vi "Bertta_v08_2.vi"() -> ()   [LabVIEW 2015]
panel:
  out "Started:":string
  in  "SHUTDOWN":bool
  in  "MASTER CONTROL":bool
  in  "Tab Control":T1(tab)
  in  "Read Seq":bool
  in  "Save Seq":bool
  in  "Configuration file":path=path "C:/Users/shresplab/Desktop/BerttaConfiguration.lvm" caption="Filename"
  in  "OK Button 2":bool
  out "Boolean":bool
  in  "User (initials)":string
  in  "Project name":string
  in  "Description":string
  out "Output file":string
  in  "OK Button":bool
  in  "Add comment":string
  out "PUMP 1":bool
  out "Target amount":dbl
  out "Scale weight":dbl
  out "Amount now":dbl
  out "Flow rate":dbl
  out "Time to target":dbl format="%<%H:%M:%S>t"
  out "Current step":dbl
  out "Target amount":dbl
  out "Amount now":dbl
  out "Tr":dbl
  out "Tj in":dbl
  out "Tj out":dbl
  out "T set":dbl
  out "Current step":i32
  out "RPM":dbl
  out "Torque 2":dbl
  out "Waveform Chart 5":dynamicdata(graph)
  out "Waveform Chart 6":dynamicdata(graph)
  out "Waveform Chart 7":dynamicdata(graph)
  in  "Tab Control 2":T2(tab)
  out "Waveform Chart 3":dynamicdata(graph)
  out "Waveform Chart 8":dynamicdata(graph)
  out "Waveform Chart 9":dynamicdata(graph)
  out "Table":string[][](table)=[["Date / time", "Flow rate, P1, g/min", "Weight, S1, g", "Amount / step, P1, g", "Step number, P1", "Total amount,P1, g ", "Tj in, C", "Tj out, C", "Tr, C", "RPM", "Torque", ""], ["11.8.2017 13.29.21", "0,000000", "423,900000", "-423,900000", "1,000000", "20,000000", "22,722972", "22,704167", "22,605956", "0,000000", "395,000000", "4,800000"], ["11.8.2017 13.29.26", "0,000000", "423,900000", "0,000000", "1,000000", "20,000000", "22,719822", "22,702434", "22,603119", "0,000000", "0,000000", "0,000000"], ["11.8.2017 13.29.31", "0,000000", "423,900000", "0,000000", "1,000000", "20,000000", "22,719034", "22,702118", "22,600441", "0,000000", "0,000000", "0,000000"], ["11.8.2017 13.29.37", "0,000000", "423,900000", "0,000000", "1,000000", "20,000000", "22,717459", "22,701015", "22,596344", "0,000000", "63,000000", "2,600000"], ["11.8.2017 13.29.42", "0,000000", "423,900000", "0,000000", "1,000000", "20,000000", "22,716829", "22,699440", "22,595242", "0,000000", "199,000000", "3,900000"], ["11.8.2017 13.29.47", "0,000000", "423,900000", "0,000000", "1,000000", "20,000000", "22,715411", "22,699282", "22,593351", "0,000000", "269,000000", "4,300000"], ["11.8.2017 13.29.52", "0,000000", "423,900000", "0,000000", "1,000000", "20,000000", "22,714466", "22,698967", "22,588624", "0,000000", "300,000000", "4,300000"], ["11.8.2017 13.29.58", "0,000000", "423,900000", "0,000000", "1,000000", "20,000000", "22,712733", "22,697234", "22,586261", "0,000000", "300,000000", "4,300000"], ["11.8.2017 13.30.03", "0,000000", "423,900000", "0,000000", "1,000000", "20,000000", "22,710370", "22,696604", "22,585315", "0,000000", "300,000000", "4,400000"], ["11.8.2017 13.30.08", "0,000000", "424,100000", "-0,200000", "1,000000", "20,000000", "22,709425", "22,696131", "22,583582", "0,000000", "300,000000", "4,300000"], ["11.8.2017 13.30.13", "0,000000", "424,200000", "-0,300000", "1,000000", "20,000000", "22,708008", "22,693925", "22,582952", "0,000000", "300,000000", "0,000000"], ["11.8.2017 13.30.18", "0,000000", "424,200000", "-0,300000", "1,000000", "20,000000", "22,706117", "22,693453", "22,583740", "0,000000", "300,000000", "4,300000"], ["11.8.2017 13.30.23", "0,000000", "424,200000", "-0,300000", "1,000000", "20,000000", "22,706747", "22,693768", "22,587048", "0,000000", "300,000000", "4,400000"], ["11.8.2017 13.30.28", "0,000000", "424,200000", "-0,300000", "1,000000", "20,000000", "22,706275", "22,694556", "22,590357", "0,000000", "300,000000", "39,100000"], ["11.8.2017 13.30.33", "0,000000", "424,200000", "-0,300000", "1,000000", "20,000000", "22,705645", "22,693925", "22,594296", "0,000000", "300,000000", "5,300000"]]
  in  "T ext / T ext 2":enum32{"External 1", "External 2"}(radio)
  out "Sensor OK":bool
  in  "T fail":dbl=20.0
  out "Boolean 12":bool
  out "Boolean 7":bool
  out "Boolean 6":bool
  out "Boolean 5":bool
  out "Boolean 4":bool
  in  "?":bool
  in  "T setpoint":dbl=20.0
  in  "Lauda port":dbl=9.0
  out "Data out":dbl
  in  "Bypass select":enum32{"Tr", "Tj"}(radio)
  in  "TempSeq":dbl[][](array[numeric])=[[20.0, 45.0, 50.0, 46.0], [46.0, 50.0, 20.0, 51.0], [20.0, 50.0, 3.0, 25.0], [20.0, 20.0, 0.0, 20.0], [20.0, 20.0, 0.0, 20.0], [20.0, 20.0, 1000.0, 20.0]]
  out "T control":dbl
  out "Tr":dbl
  out "Tj in":dbl
  out "Tj out":dbl
  out "DT":dbl
  out "Elapsed":i32
  in  "PAUSE":bool
  out "Boolean 19":bool
  in  "Reset":bool
  in  "Treshold (Tset)":dbl=1.0
  in  "Tmax":dbl=140.0
  in  "Tmin":dbl=20.0
  out "Current step":i32
  out "Tset":dbl
  out "Waveform Chart":dynamicdata(graph)
  out "T external 2":dbl
  in  "Ring":u16(ring) items=["SCALE 1", "SCALE 2", "SCALE 3"]
  out "Data out":dbl
  out "Port":i32=10
  in  "Radio Buttons":enum32{"Reglo Digital", "Reglo Analog", "PAM"}(radio)
  out "Speed":dbl
  out "mA":dbl format="%#_2g"
  in  "Port":i32=15
  out "RPM":dbl format="%#_2g"
  out "Boolean 18":bool
  out "Boolean 17":bool
  out "Boolean 16":bool
  out "Boolean 15":bool
  out "Boolean 14":bool
  out "Boolean 13":bool
  out "Boolean 11":bool
  out "Boolean 10":bool
  out "Boolean 9":bool
  out "Boolean 8":bool
  in  "PumpSeq":dbl[][](array[numeric])=[[3.0, 3.0, 7.0], [2.0, 2.0, 2.0], [4.0, 2.0, 100.0], [0.0, 0.0, 0.0], [0.0, 0.0, 0.0], [0.0, 0.0, 0.0], [0.0, 0.0, 0.0], [0.0, 0.0, 0.0], [0.0, 0.0, 0.0], [0.0, 0.0, 0.0], [0.0, 1.0, 0.0]]
  in  "?":bool
  out "Flow rate (g/min)":dbl
  out "Time (min)":dbl
  out "Target (g)":dbl
  out "Scale reading":dbl
  out "Step amount now":dbl
  out "Time to target":dbl format="%<%H:%M:%S>t"
  in  "Grams / min":dbl
  out "Waveform Chart 2":dynamicdata(graph)
  in  "?":bool
  out "Total amount now":dbl
  out "Total time":dbl
  out "Total amount target":dbl
  out "Boolean 20":bool
  in  "Reset 2":bool
  in  "Bypass select 2":enum32{"Remote", "Manual"}(radio)
  in  "Port":dbl=13.0
  out "RPM":dbl
  out "Torque":dbl
  in  "Set RPM":dbl(slide) scale=0.0..500.0
  out "Waveform Chart 4":dynamicdata(graph)
  out "DAQ 9217 (PT100)":errorcluster
  # "PUMP & SCALE 1"
  # "STEP"
  # "TOTAL"
  # "Tinit     >    Tset       Min. time      Tfail"
  # "Manual control / end of sequence"
  # "Manual control"
  # "Secondary temperature sensor"
  # "Device communication"
  # "Grams    /   min"
  # "End of sequence"
  # "Manual control"
  # "Device communication"
  # "Pump configuration"
  # "Scale configuration"
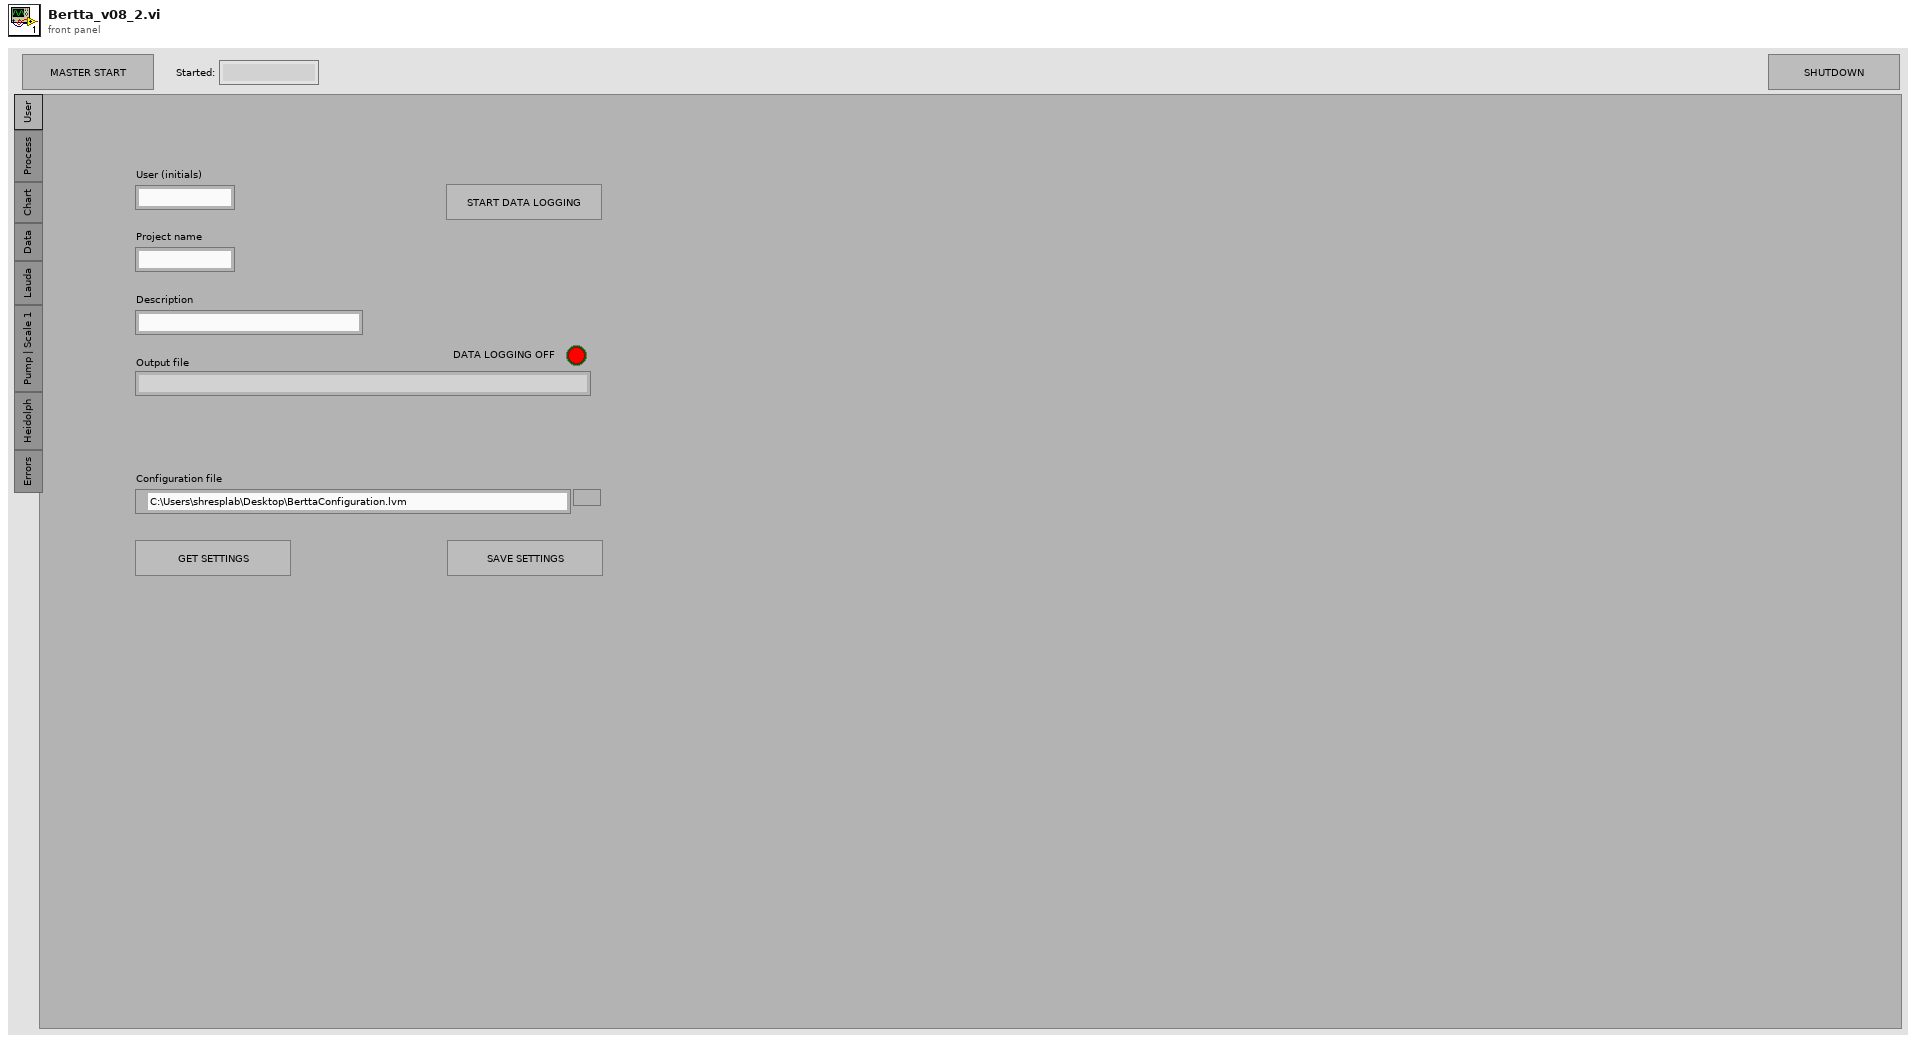
[diagram p1: front panel]
types:
  T1 = enum32{"User", "Process", "Chart", "Data", "Lauda", "Pump | Scale 1", "Heidolph", "Errors"}
  T2 = enum32{"Temperatures", "Scale / Pump 1", "RPM / torque"}
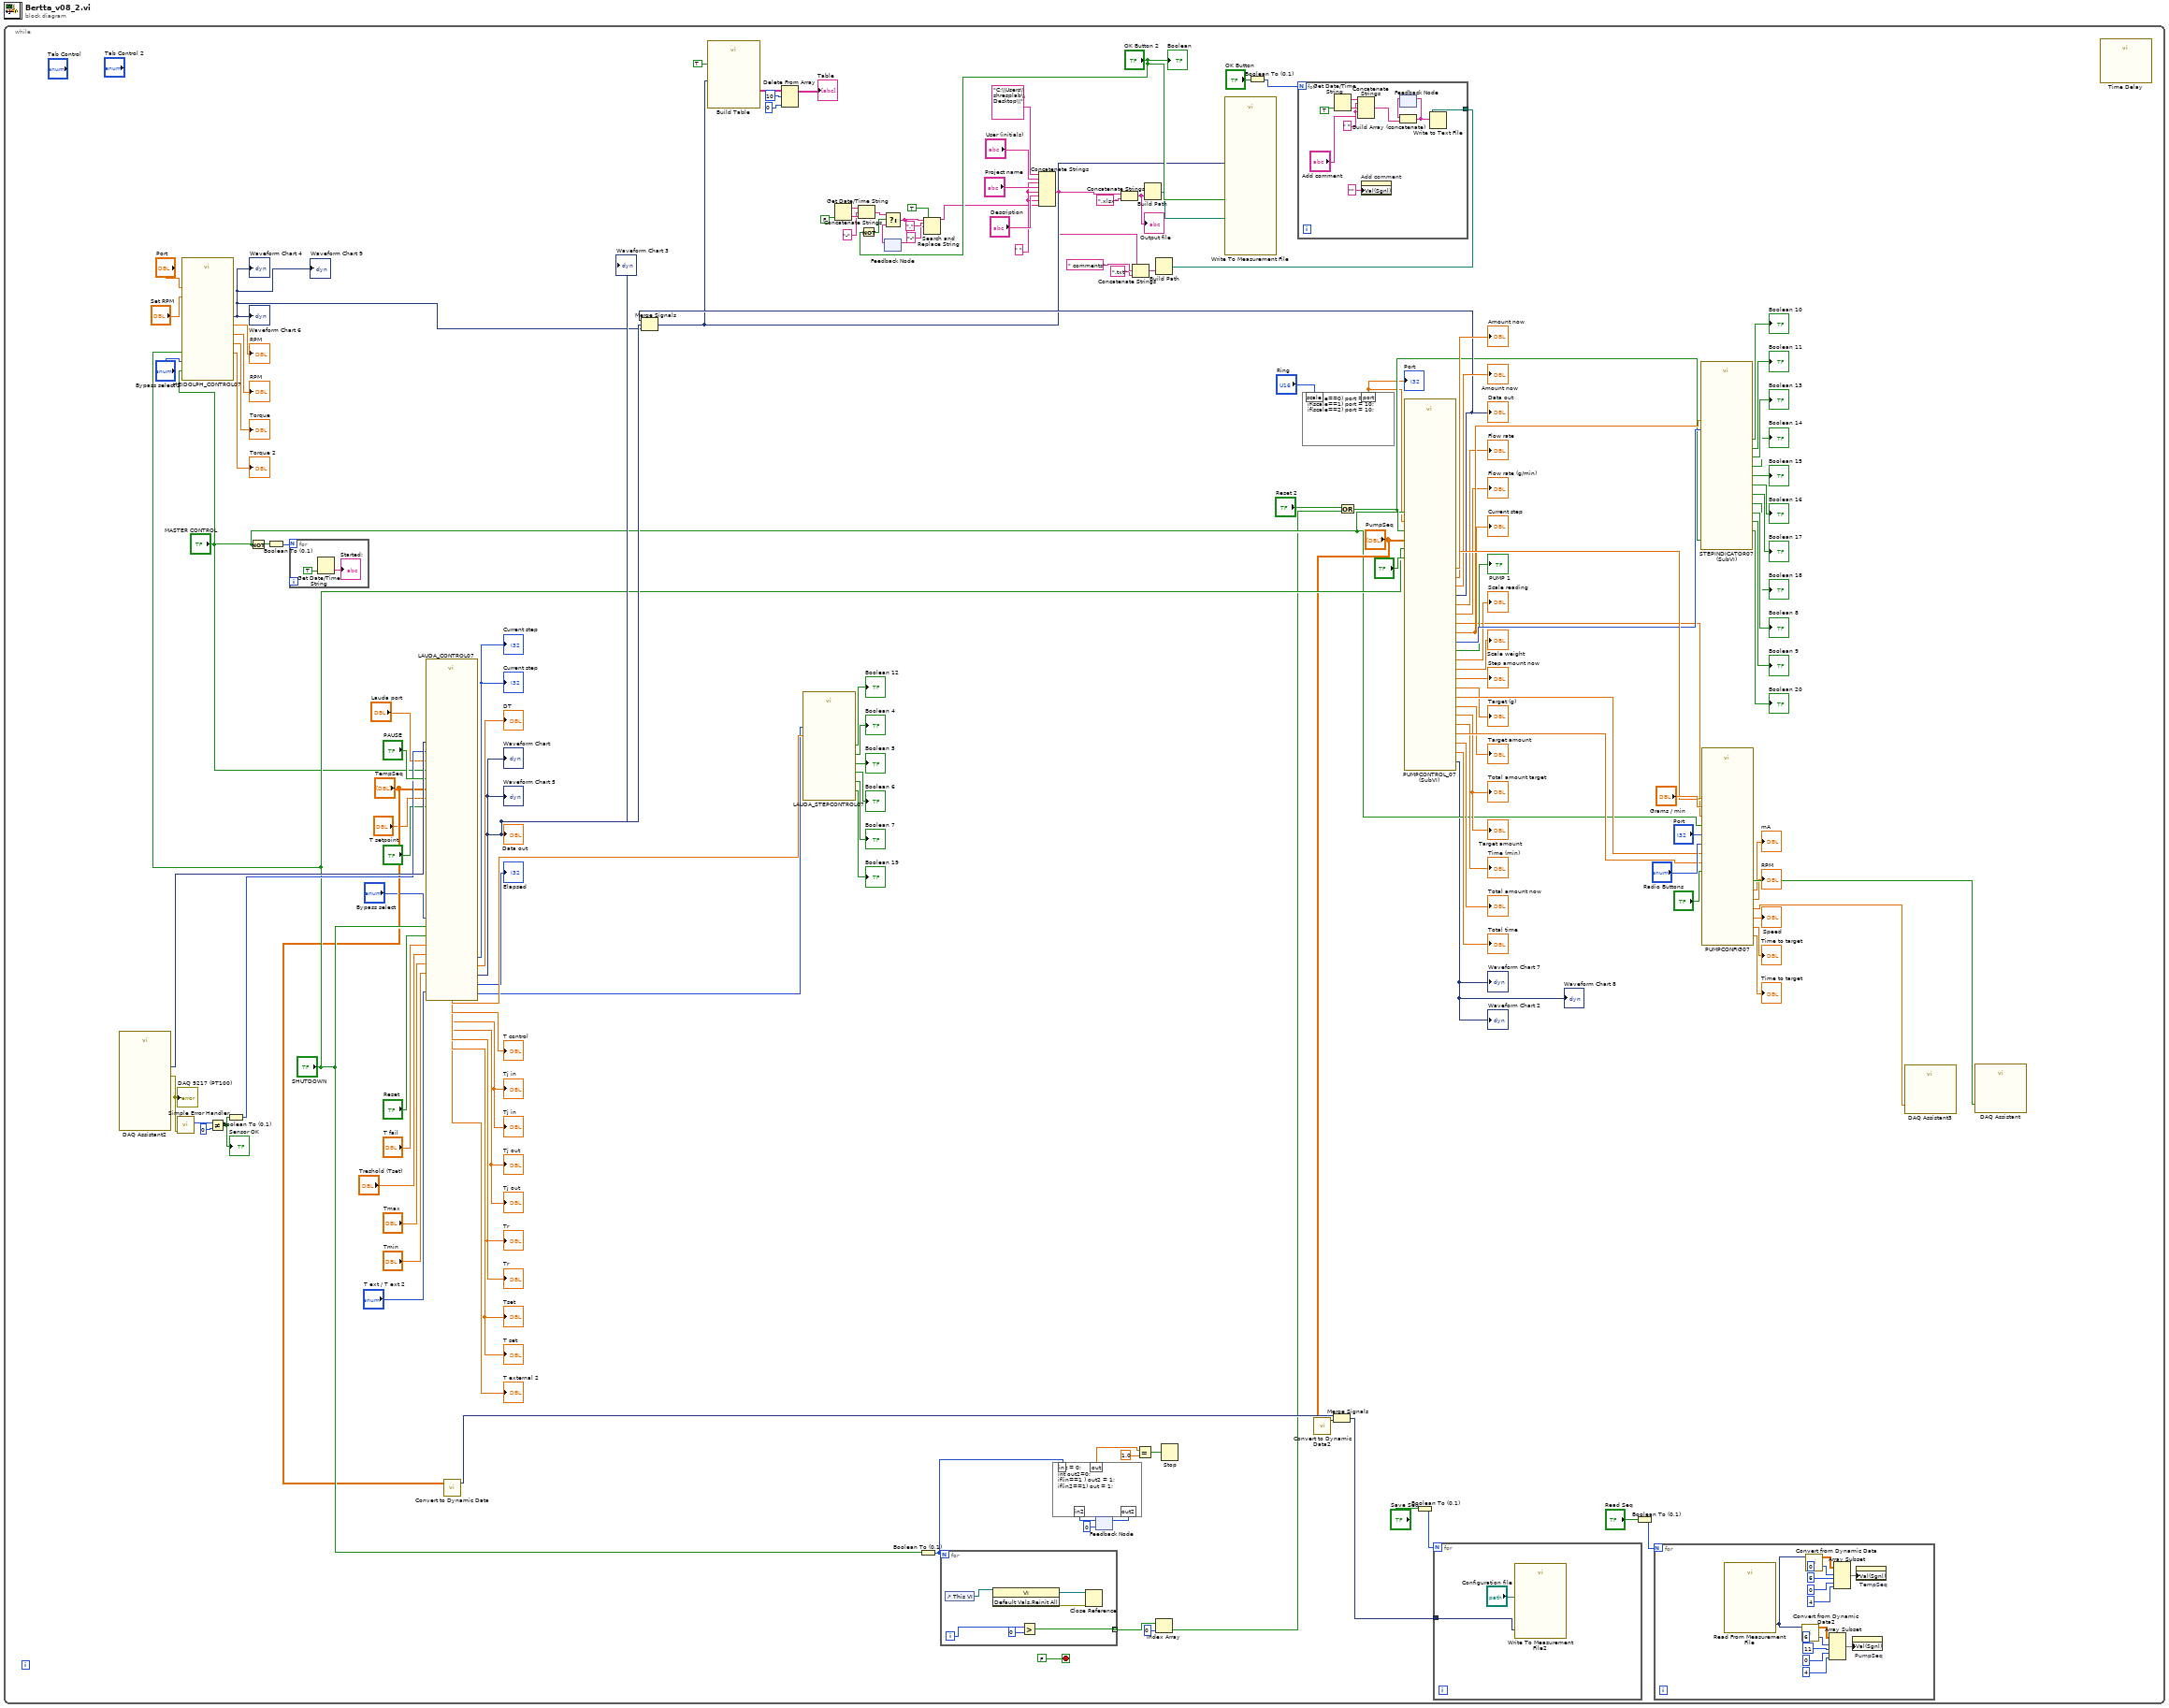
[diagram p0: block diagram]
diagram:
  n1 = while {
    stop <- FALSE stop-if-true
    w81 = " "
    n2 = call "DAQ Assistant2"() -> ("data"=w144:dynamicdata, "error out"=w88:errorcluster)  [unwired: 17 in, 1 out]
    "DAQ 9217 (PT100)" <- w88
    n3 = call <vilib>:"Simple Error Handler.vi"("error in (no error)"=w88) -> ("code out"=w87:i32)  [unwired: 4 in, 4 out]
    n4 = call "HEIDOLPH_CONTROL07.vi"("master"="MASTER CONTROL", "shutdown"="SHUTDOWN", "Bypass select"="Bypass select 2", "Set RPM"="Set RPM", "Device port"="Port") -> ("Dynamic Data"=w93:dynamicdata, "RPM"=→"RPM":dbl, "RPM 2"=→"RPM":dbl, "Torque"=→"Torque":dbl, "Torque 2"=→"Torque 2":dbl)  [unwired: 2 in]
    "Waveform Chart 4" <- w93
    "Waveform Chart 6" <- w93
    "Waveform Chart 9" <- w93
    n5 = Not Equal?(x=w87, y=0) -> (x != y?=w51:bool)
    "Sensor OK" <- w51
    n6 = Boolean To (0,1)(Boolean=w51) -> (0, 1=w85:i16)
    n7 = Not(x="MASTER CONTROL") -> (.not. x?=w69:bool)
    n8 = Boolean To (0,1)(Boolean=w69) -> (0, 1=w70:i16)
    n9 = for {
      N: w70 -> [_]
      n10 = Get Date/Time String(want seconds? (F)=TRUE) -> (time string=→"Started:":string)  [unwired: 2 in, 1 out]
    }
    n11 = call "LAUDA_CONTROL07.vi"("Bypass"="?", "PAUSE"="PAUSE", "data"=w144, "Seq"="TempSeq", "Lauda port"="Lauda port", "Tbypass"="T setpoint", "Treshold"="Treshold (Tset)", "Bypass select"="Bypass select", "err"=w85, "Shutdown"="SHUTDOWN", "Master Start"="MASTER CONTROL", "Reset"="Reset", "Tfail (manual)"="T fail", "Tmax"="Tmax", "T ext / T ext 2"="T ext / T ext 2", "Tmin"="Tmin") -> ("Tj in"=→"Tj in" →"Tj in":dbl, "DT"=→"DT":dbl, "Tj out"=→"Tj out" →"Tj out":dbl, "Tset"=→"Tset" →"T set":dbl, "Dynamic Data"=w95:dynamicdata, "T ext 2"=→"T external 2":dbl, "Numeric"=w73:i16, "Numeric 2"=w149:dbl, "T control"=→"T control":dbl, "Current step"=→"Current step" →"Current step":i32, "Elapsed"=→"Elapsed":i32, "Tr"=→"Tr" →"Tr":dbl)
    "Waveform Chart 3" <- w95
    "Waveform Chart" <- w95
    "Data out" <- w95
    "Waveform Chart 5" <- w95
    n12 = call "Convert to Dynamic Data"("2D Array"="TempSeq") -> ("Dynamic Data Type"=w61:dynamicdata)  [unwired: 3 in]
    n13 = call "LAUDA_STEPCONTROL07.vi"("Numeric 2"=w149, "Numeric"=w73) -> ("Boolean 13"=→"Boolean 19":bool, "Boolean 6"=→"Boolean 6":bool, "Boolean 5"=→"Boolean 5":bool, "Boolean 4"=→"Boolean 4":bool, "Boolean 7"=→"Boolean 7":bool, "Boolean 12"=→"Boolean 12":bool)  [unwired: 4 in]
    n14 = Get Date/Time String(want seconds? (F)=FALSE) -> (date string=w35:string, time string=w30:string)  [unwired: 2 in]
    n15 = Concatenate Strings(w35, "-" ("string"), w30) -> (w34:string)
    n16 = Not(x="OK Button 2") -> (.not. x?=w31:bool)
    n17 = feedback #1() -> (w33:string)  [unwired: 1 in]
    n18 = Select(t=w34, s=w31, f=w33) -> (s? t:f=w26:string)
    n19 = feedback-in #1(w26) -> ()
    n20 = Boolean To (0,1)(Boolean="SHUTDOWN") -> (0, 1=w4:i16)
    n21 = Search and Replace String(replace all?=TRUE ("replace all? (F)"), input string=w26, search string=".", replace string="-" ("replace string (\"\")")) -> (result string=w25:string)  [unwired: 4 in, 3 out]
    n22 = for {
      N: w4 -> [_]
      tunnel: [w176] -> w64 mode=indexing
      i -> [w178]
      n23 = control-ref of="This VI"() -> (w181:refnum<vi>)
      n24 = invoke class="VI" method="Default Vals.Reinit All"(reference=w181) -> (reference out=w179:refnum<vi>, error out=w180:errorcluster)  [unwired: 2 in, 1 out]
      n25 = Greater?(x=w178, y=0) -> (0:w176:bool)
      n26 = Close Reference(reference=w179, error in (no error)=w180) -> ()  [unwired: 1 out]
    }
    n27 = Concatenate Strings("C:\\Users\\shresplab\\Desktop\\", "User (initials)", w81, "Project name", w81, "Description", w81, w25) -> (w15:string)
    n28 = feedback #2(0) -> (w2:i32)
    n29 = formula code="out = 0;\nint out2=0;\nif(in==1 ) out2 = 1;\nif(in2==1) out = 1;"("in"=w4, "in2"=w2) -> ("out"=w7:dbl, "out2"=w3:i32)
    n30 = feedback-in #2(w3) -> ()
    n31 = Concatenate Strings(w15, ".xlsx") -> (w18:string)
    "Output file" <- w18
    n32 = Concatenate Strings(w15, " comments" ("string"), ".txt" ("string")) -> (w12:string)
    n33 = Equal?(x=w7, y=1.0) -> (x = y?=w6:bool)
    n34 = Build Path(name or relative path=w18) -> (appended path=w16:path)  [unwired: 1 in]
    n35 = Index Array(array=w64, index=0) -> (element=w5:bool)
    n36 = Build Path(name or relative path=w12) -> (appended path=w11:path)  [unwired: 1 in]
    n37 = Stop(stop? (T)=w6) -> ()
    n38 = Boolean To (0,1)(Boolean="OK Button") -> (0, 1=w10:i16)
    n39 = for {
      N: w10 -> [_]
      tunnel: w11 -> [w153]
      w157 = " " ("string")
      n40 = Get Date/Time String(want seconds? (F)=TRUE) -> (date string=w160:string, time string=w158:string)  [unwired: 2 in]
      n41 = Concatenate Strings(w160, w157, w158, w157, "Add comment") -> (w156:string)
      n42 = property on="Add comment" class="Str"("Val(Sgnl)"="" ("Value (Signaling)")) -> ()  [unwired: 2 in, 2 out]
      n43 = feedback #3() -> (w155:string[])  [unwired: 1 in]
      n44 = Build Array (concatenate)(w155, w156) -> (w154:string[])
      n45 = feedback-in #3(w154) -> ()
      n46 = Write to Text File(file (use dialog)=w153, text=w154) -> ()  [unwired: 2 in, 3 out]
    }
    n47 = formula code="if(scale==0) port = 10;\nif(scale==1) port = 10;\nif(scale==2) port = 10;"("scale"="Ring") -> ("port"=w39:dbl)
    "Port" <- w39
    n48 = call "Convert to Dynamic Data2"("2D Array"="PumpSeq") -> ("Dynamic Data Type"=w59:dynamicdata)  [unwired: 3 in]
    n49 = Merge Signals(w61, w59) -> (w58:dynamicdata)
    n50 = Or(x="Reset 2", y=w5) -> (x .or. y?=w50:bool)
    n51 = call "PUMPCONTROL_07 (SubVI).vi"("Port"=w39, "Pause"="MASTER CONTROL", "Master start"="?", "shutdown"="SHUTDOWN", "Seq in"="PumpSeq", "reset"=w50) -> ("Amount now"=→"Amount now":dbl, "Amount now 2"=→"Amount now":dbl, "Flow rate out"=w76:dbl, "Step amount now"=→"Step amount now":dbl, "Total amount now"=→"Total amount now":dbl, "Total time"=→"Total time":dbl, "Numeric 2"=w140:i16, "PUMP 1"=→"PUMP 1":bool, "Numeric"=w136:dbl, "Flow rate"=→"Flow rate":dbl, "Dynamic Data"=w94:dynamicdata, "Target amount"=→"Target amount":dbl, "Time (min) 2"=w141:dbl, "Target amount 2"=→"Total amount target" →"Target amount":dbl, "Scale reading"=→"Scale reading":dbl, "Flow rate (g/min)"=→"Flow rate (g/min)":dbl, "Target (g) 2"=w142:dbl, "Target (g)"=→"Target (g)":dbl, "Time (min)"=→"Time (min)":dbl, "Waveform Chart 2"=→"Waveform Chart 2" →"Waveform Chart 7" →"Waveform Chart 8":dynamicdata, "Scale weight"=→"Scale weight":dbl, "Amount (g)"=w143:dbl)
    "Current step" <- w136
    "Data out" <- w94
    n52 = Merge Signals(w94, w95, w93) -> (w22:dynamicdata)
    n53 = call "Build Table"("Include time data"=TRUE, "Signals"=w22) -> ("Table"=w21:string[][])  [unwired: 3 in, 6 out]
    n54 = Delete From Array(array=w21, length=10, index (col)=0 ("index (row)")) -> (array with subset deleted=→"Table":string[][])  [unwired: 1 in, 1 out]
    n55 = call "Write To Measurement File"("Signals"=w22, "Enable"="OK Button 2", "Filename"=w16) -> ()  [unwired: 14 in, 3 out]
    n56 = Boolean To (0,1)(Boolean="Save Seq") -> (0, 1=w57:i16)
    n57 = for {
      N: w57 -> [_]
      tunnel: w58 -> [w175]
      n58 = call "Write To Measurement File2"("Signals"=w175, "Filename"="Configuration file") -> ()  [unwired: 15 in, 3 out]
    }
    n59 = Boolean To (0,1)(Boolean="Read Seq") -> (0, 1=w54:i16)
    n60 = for {
      N: w54 -> [_]
      n61 = call "Read From Measurement File"() -> ("Signals"=w163:dynamicdata)  [unwired: 6 in, 5 out]
      n62 = call "Convert from Dynamic Data2"("Dynamic Data Type"=w163) -> ("Array"=w162:dbl[][])  [unwired: 3 in]
      n63 = call "Convert from Dynamic Data"("Dynamic Data Type"=w163) -> ("Array"=w171:dbl[][])  [unwired: 3 in]
      n64 = Array Subset(array=w162, index (row)=6 ("index"), length (row)=11 ("length"), index (col)=0 ("index"), length (col)=4 ("length")) -> (w161:dbl[][])
      n65 = Array Subset(array=w171, index (row)=0 ("index"), length (row)=6 ("length"), index (col)=0 ("index"), length (col)=4 ("length")) -> (w168:dbl[][])
      n66 = property on="PumpSeq" class="Arr (strict)"("Val(Sgnl)"=w161) -> ()  [unwired: 2 in, 2 out]
      n67 = property on="TempSeq" class="Arr (strict)"("Val(Sgnl)"=w168) -> ()  [unwired: 2 in, 2 out]
    }
    n68 = call "STEPINDICATOR07 (SubVI).vi"("Numeric"=w136, "Numeric 2"=w140, "Reset"=w50) -> ("Boolean 18"=→"Boolean 18":bool, "Boolean 8"=→"Boolean 8":bool, "Boolean 9"=→"Boolean 9":bool, "Boolean 17"=→"Boolean 17":bool, "Boolean 10"=→"Boolean 10":bool, "Boolean 16"=→"Boolean 16":bool, "Boolean 11"=→"Boolean 11":bool, "Boolean 15"=→"Boolean 15":bool, "Boolean 14"=→"Boolean 14":bool, "Boolean 13"=→"Boolean 13":bool, "Boolean 19"=→"Boolean 20":bool)  [unwired: 2 in]
    n69 = call "PUMPCONFIG07.vi"(0:"?", "Radio Buttons"="Radio Buttons", "Bypass (g/min)"="Grams / min", "Target (g) in"=w142, "Amount (g)"=w143, "Time (min) in"=w141, "Flow rate in"=w76, "OK Button"="MASTER CONTROL", "Port"="Port") -> ("Time to target 2"=→"Time to target":dbl, "Time to target"=→"Time to target":dbl, "mA"=→"mA":dbl, "signal"=w147:dbl, "Speed"=→"Speed":dbl, "RPM"=→"RPM":dbl, "Array"=w148:bool[])
    n70 = call "DAQ Assistant3"("data"=w147) -> ()  [unwired: 17 in, 2 out]
    n71 = call "DAQ Assistant"("data"=w148) -> ()  [unwired: 17 in, 2 out]
    n72 = call "Time Delay"() -> ()  [unwired: 11 in, 1 out]
    "Boolean" <- "OK Button 2"
  }
